vi "Paths for seq. shot v0.3.vi"(4 "Base Filename Prefix":string="MyData", 5 "Default Path":path=path "/Volumes/DATA", 6 "FieldRamp Parameters":dbl[][](array[numeric])=[[0.0, 30.0, 1.0, 400.0], [30.0, 0.0, -1.0, 400.0], [0.0, -30.0, -1.0, 400.0], [-30.0, 0.0, 1.0, 400.0], [0.0, 30.0, 0.5, 200.0], [30.0, 0.0, -0.5, 200.0]] step=1.0 format="%.2f", 7 "RampIndexSelect":bool[](array[boolean])=[TRUE, TRUE, FALSE, FALSE, FALSE, FALSE]) -> (0 "FilePrefix for the sequences":string[](array[string]), 1 "Default Path for the sequences":path[](array[path]), 2 "FieldRamp Parameters out":dbl[][](array[numeric])=[[0.0, 30.0, 1.0, 400.0], [30.0, 0.0, -1.0, 400.0], [0.0, -30.0, -1.0, 400.0], [-30.0, 0.0, 1.0, 400.0], [0.0, 30.0, 0.5, 200.0], [30.0, 0.0, -0.5, 200.0]] step=1.0 format="%.2f", 3 "RampIndexSelect out":bool[](array[boolean])=[TRUE, TRUE, FALSE, FALSE, FALSE, FALSE])   [LabVIEW 2025]
doc: "Author: Scott Hannahs <sth@magnet.fsu.edu>\n\nThis software is licensed for use under the “MIT License\"\nCopyright (c) 2025 Scott Hannahs, sth@sth@magnet.sthnet.net\n\nPermission is hereby granted, free of charge, to any person obtaining a copy of this software and associated documentation files (the \"Software\"), to deal in the Software without restriction, including without limitation the rights to use, copy, modify, merge, publish, distribute, sublicense, and/or sell copies of the Software, and to permit persons to whom the Software is furnished to do so, subject to the following conditions: The above copyright notice and this permission notice shall be included in all copies or substantial portions of the Software.\n\nTHE SOFTWARE IS PROVIDED \"AS IS\", WITHOUT WARRANTY OF ANY KIND, EXPRESS OR IMPLIED, INCLUDING BUT NOT LIMITED TO THE WARRANTIES OF MERCHANTABILITY, FITNESS FOR A PARTICULAR PURPOSE AND NONINFRINGEMENT. IN NO EVENT SHALL THE AUTHORS OR COPYRIGHT HOLDERS BE LIABLE FOR ANY CLAIM, DAMAGES OR OTHER LIABILITY, WHETHER IN AN ACTION OF CONTRACT, TORT OR OTHERWISE, ARISING FROM, OUT OF OR IN CONNECTION WITH THE SOFTWARE OR THE USE OR OTHER DEALINGS IN THE SOFTWARE."
panel:
  in  "All Sequences":bool
  in  "Return":bool=TRUE
  in  "Diff Prefix?":bool=TRUE caption="Same Prefix"
  in  "FilePrefix":string[](array[string])=["", "", "", "", "", ""]
  in  "Sub Folder?":bool=TRUE caption="No Sub Folder"
  in  "SubfolderName":string[](array[string])=["", "", "", "", "", ""]
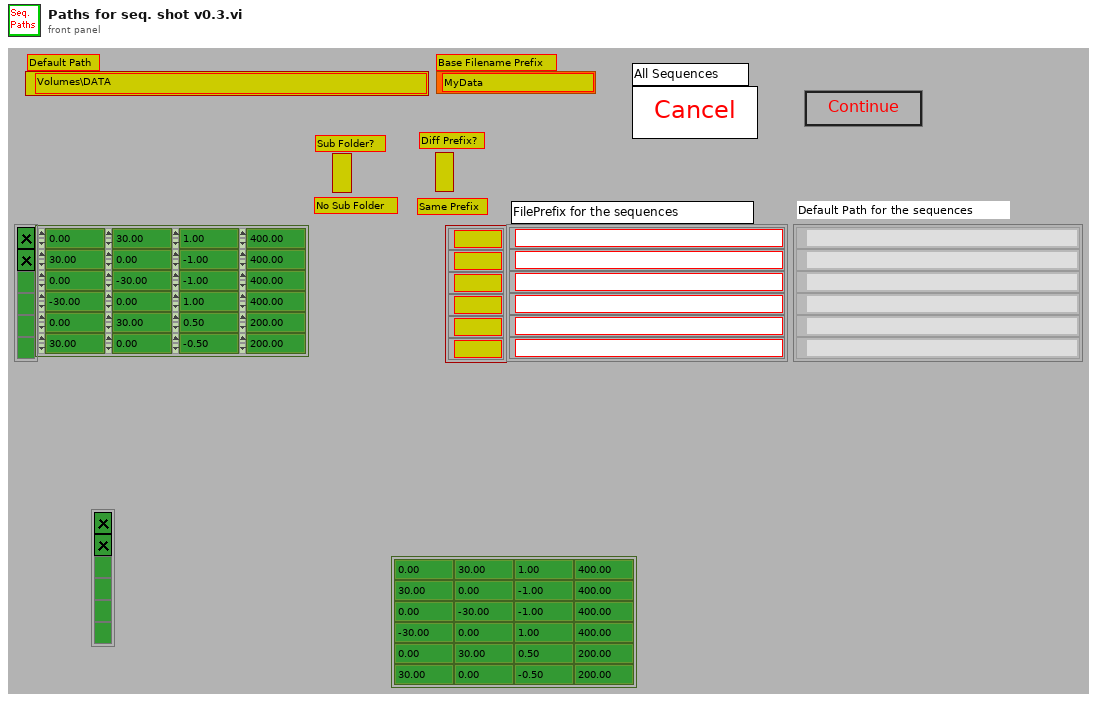
[diagram p1: front panel]
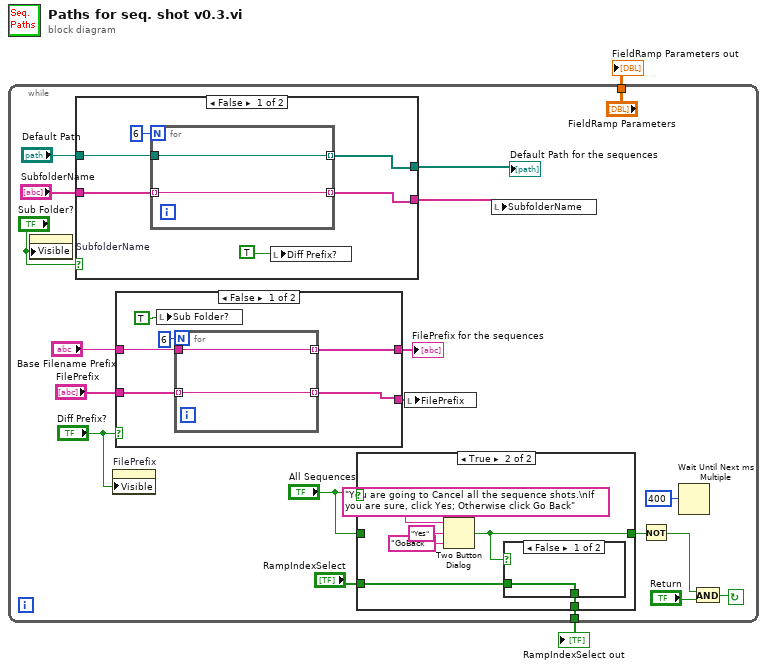
[diagram p0: block diagram]
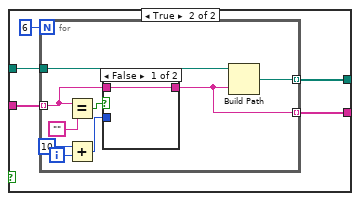
[diagram p2: hidden frame]
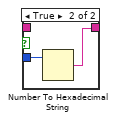
[diagram p3: hidden frame]
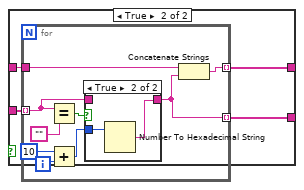
[diagram p4: hidden frame]
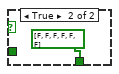
[diagram p7: hidden frame]
diagram:
  n1 = while {
    tunnel: [w20] -> w1
    tunnel: ["FieldRamp Parameters"] -> w2
    stop <- w14 continue-if-true
    n2 = property on="SubfolderName" class="Arr (strict)"("Visible"="Sub Folder?") -> ()  [unwired: 2 in, 2 out]
    n3 = case shown="False" "Sub Folder?" {
      tunnel: "SubfolderName" -> [w23 w33]
      tunnel: "Default Path" -> [w25 w32]
      tunnel: [w24 w31] -> w10
      tunnel: [w22 w30] -> w9
      frame False {
        n4 = for {
          N: 6 -> [_]
          tunnel: [w29] -> w24 mode=indexing
          tunnel: w25 -> [w29]
          tunnel: [w28] -> w22 mode=indexing
          tunnel: w23 -> [w28] mode=indexing
        }
        n5 = local write "Diff Prefix?"(TRUE ("Diff Prefix?")) -> ()
      }
      frame True {
        n6 = for {
          N: 6 -> [_]
          tunnel: w33 -> [w41] mode=indexing
          tunnel: w32 -> [w40]
          tunnel: [w39] -> w31 mode=indexing
          tunnel: [w36] -> w30 mode=indexing
          i -> [w38]
          n7 = Equal?(x=w41, y="") -> (x = y?=w42:bool)
          n8 = Add(x=10, y=w38) -> (x+y=w35:i32)
          n9 = case shown="False" w42 {
            tunnel: w41 -> [w44 _]
            tunnel: [w44 w45] -> w36
            tunnel: w35 -> [_ w46]
            frame False {
            }
            frame True {
              n10 = Number To Hexadecimal String(2:w46) -> (0:w45:string)  [unwired: 1 in]
            }
          }
          n11 = Build Path(base path=w40, name or relative path=w36) -> (appended path=w39:path)
        }
      }
    }
    "Default Path for the sequences" <- w10
    n12 = property on="FilePrefix" class="Arr (strict)"("Visible"="Diff Prefix?") -> ()  [unwired: 2 in, 2 out]
    n13 = case shown="False" "Diff Prefix?" {
      tunnel: "Base Filename Prefix" -> [w50 w56]
      tunnel: [w49 w55] -> w7
      tunnel: "FilePrefix" -> [w48 w58]
      tunnel: [w47 w57] -> w5
      frame False {
        n14 = local write "Sub Folder?"(TRUE ("Sub Folder?")) -> ()
        n15 = for {
          N: 6 -> [_]
          tunnel: w50 -> [w54]
          tunnel: [w54] -> w49 mode=indexing
          tunnel: w48 -> [w53] mode=indexing
          tunnel: [w53] -> w47 mode=indexing
        }
      }
      frame True {
        n16 = for {
          tunnel: w58 -> [w65] mode=indexing
          tunnel: [w60] -> w57 mode=indexing
          tunnel: w56 -> [w61]
          tunnel: [w59] -> w55 mode=indexing
          i -> [w64]
          n17 = Equal?(x=w65, y="") -> (x = y?=w66:bool)
          n18 = Add(x=10, y=w64) -> (x+y=w62:i32)
          n19 = case shown="True" w66 {
            tunnel: w65 -> [w68 _]
            tunnel: [w68 w69] -> w60
            tunnel: w62 -> [_ w70]
            frame False {
            }
            frame True {
              n20 = Number To Hexadecimal String(2:w70) -> (0:w69:string)  [unwired: 1 in]
            }
          }
          n21 = Concatenate Strings(w61, w60) -> (w59:string)
        }
      }
    }
    "FilePrefix for the sequences" <- w7
    n22 = case shown="True" "All Sequences" {
      tunnel: [w71 w75] -> w17
      tunnel: [w72 w74] -> w20
      tunnel: "RampIndexSelect" -> [w72 w73]
      tunnel: "All Sequences" -> [w71 _]
      frame False {
      }
      frame True {
        n23 = Two Button Dialog(message="You are going to Cancel all the sequence shots.\nIf you are sure, click Yes; Otherwise click Go Back", 1:"GoBack" ("F button name (\"Cancel\")"), 2:"Yes" ("T button name (\"OK\")")) -> (T button?=w75:bool)
        n24 = case shown="False" w75 {
          tunnel: [w79 bool[] [FALSE, FALSE, FALSE, FALSE, FALSE, FALSE] ("RampIndexSelect out")] -> w74
          tunnel: w73 -> [w79 _]
          frame False {
          }
          frame True {
          }
        }
      }
    }
    n25 = local write "FilePrefix"(w5) -> ()
    n26 = local write "SubfolderName"(w9) -> ()
    n27 = Not(x=w17) -> (.not. x?=w15:bool)
    n28 = Wait Until Next ms Multiple(millisecond multiple=u32 400) -> ()  [unwired: 1 out]
    n29 = And(x=w15, y="Return") -> (x .and. y?=w14:bool)
  }
  "FieldRamp Parameters out" <- w2
  "RampIndexSelect out" <- w1
